vi "Font Scale from Required Height.vi"   [LabVIEW 2020, in "image.lvlib"]
uses:
  image.lvlib
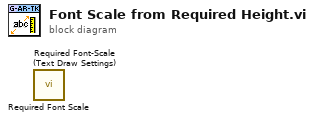
[diagram p0: block diagram]
diagram:
  n1 = call "Required Font Scale.vi"() -> ()  [unwired: 10 in, 2 out]
  n2 = call "Required Font-Scale (Text Draw Settings).vi"() -> ()  [unwired: 10 in, 2 out]
